vi "tempTest.vi"() -> ()   [LabVIEW 2019]
uses:
  <vilib>/JDP Science/JSONtext/JSONtext.lvlib
panel:
  out "Item Names":string[][](array[string])
  in  "Context":string[](array[string])=["{\"NI_ChannelName\":\"Sine\",\"NI_ExpIsRelativeTime\":true,\"NI_ExpStartTimeStamp\":\"2020-11-05T18:59:47.228Z\",\"NI_ExpTimeStamp\":\"2020-11-05T18:59:47.228Z\",\"NI_ExpXDimension\":\"t\",\"wf_increment\":0.001,\"wf_start_time\":\"1904-01-01T00:00:00.000Z\",\"wf_samples\":500,\"NI_DataType\":11}", "{\"NI_ChannelName\":\"Sine\",\"NI_ExpIsRelativeTime\":true,\"NI_ExpStartTimeStamp\":\"2020-11-05T18:59:46.890Z\",\"NI_ExpTimeStamp\":\"2020-11-05T18:59:46.890Z\",\"NI_ExpXDimension\":\"t\",\"Vendor\":\"NI\",\"Station Number\":10,\"wf_increment\":0.001,\"wf_start_time\":\"1904-01-01T00:00:00.000Z\",\"wf_samples\":500,\"NI_DataType\":11}"]
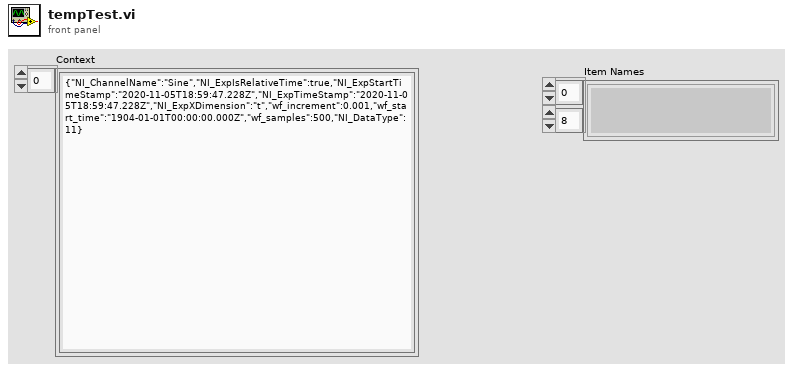
[diagram p1: front panel]
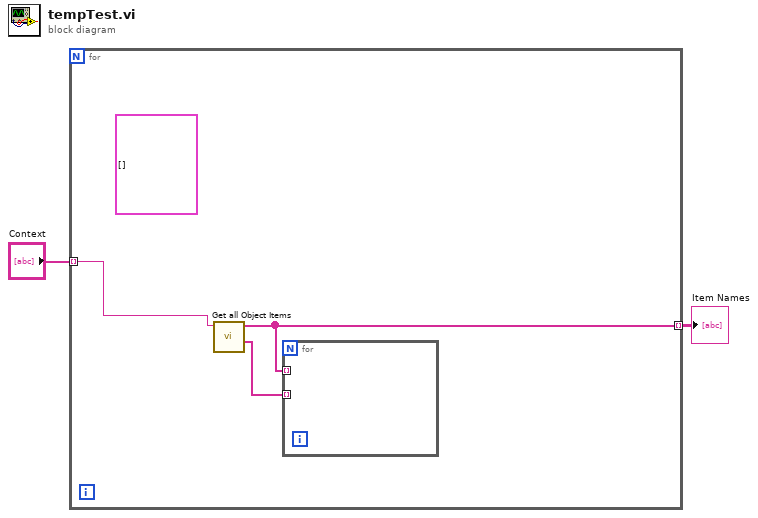
[diagram p0: block diagram]
diagram:
  n1 = for {
    tunnel: "Context" -> [w5] mode=indexing
    tunnel: [w3] -> w1 mode=indexing
    (unwired) cluster{"Name":string, "Value":variant}[] []
    n2 = call <vilib>:"Get all Object Items.vi"("JSON"=w5) -> ("<JSON>"=w4:string[], "Item Names"=w3:string[])  [unwired: 7 in, 2 out]
    n3 = for {
      tunnel: w4 -> [_] mode=indexing
      tunnel: w3 -> [_] mode=indexing
    }
  }
  "Item Names" <- w1
